vi "WriteToGlobalsFromNT.vi"() -> ()   [LabVIEW 2019]
uses:
  <vilib>/Rock Robotics/Network Tables/NT Read String Array.vi
  CalibrationsGlobalVariables.vi
panel:
  in  "ControlPanelArray":string[](array[string])=["Spinwheel_Throttle", "time_to_run"]
  in  "MagazineArray":string[](array[string])=["Top_IR_Threshold", "Top_Middle_IR_Threshold", "Bottom_Middle_IR_Threshold", "Bottom_IR_Threshold", "Loading_Speed", "Firing_Speed", "Unjam_Speed", "Max_Magazine_Speed"]
  in  "IntakeArray":string[](array[string])=["retract_delay(ms)", "extend_delay(ms)", "Intake Input", "Hopper Input", "Intake_Speed"]
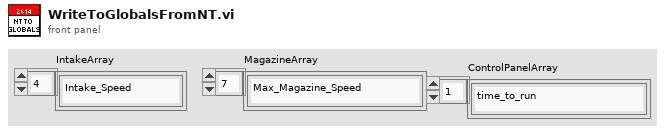
[diagram p1: front panel]
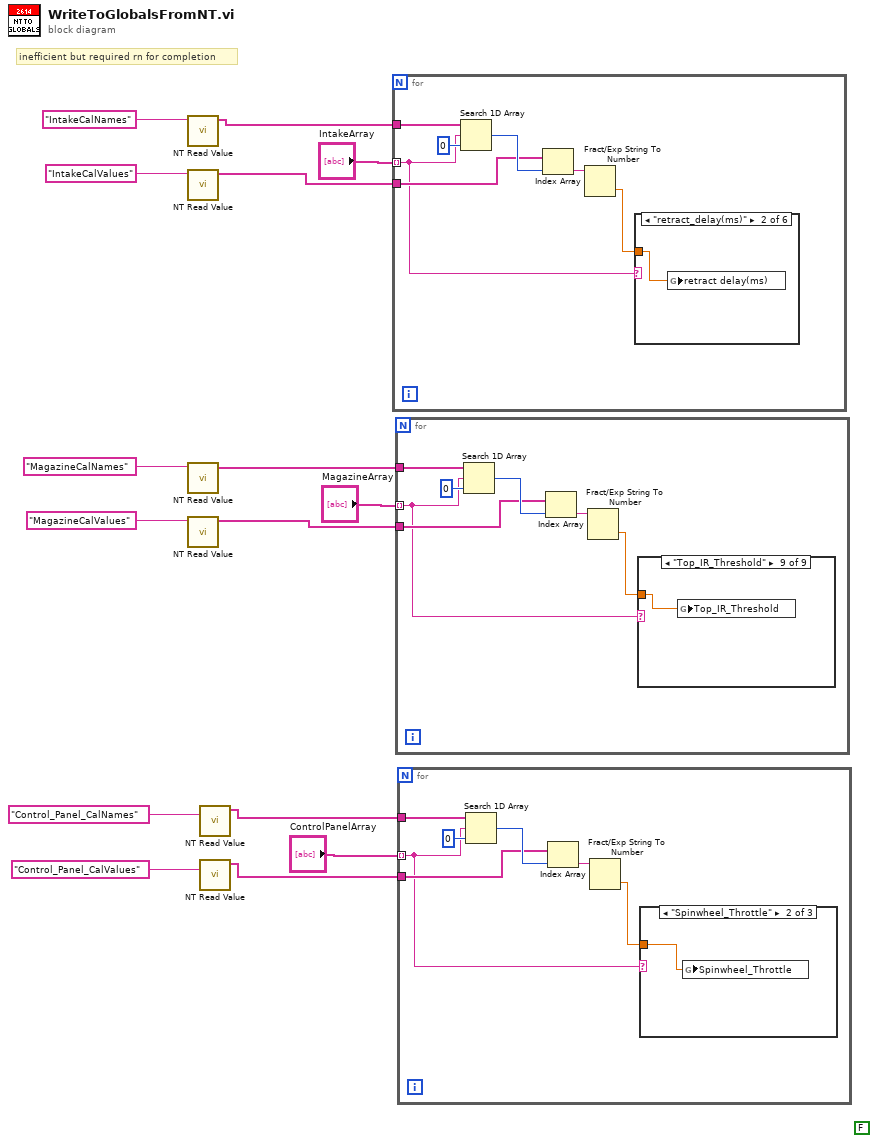
[diagram p0: block diagram]
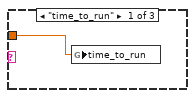
[diagram p2: hidden frame]
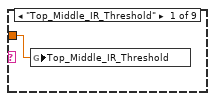
[diagram p4: hidden frame]
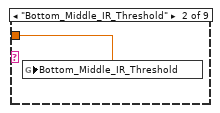
[diagram p5: hidden frame]
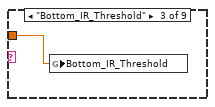
[diagram p6: hidden frame]
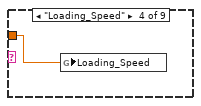
[diagram p7: hidden frame]
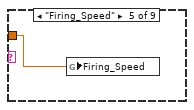
[diagram p8: hidden frame]
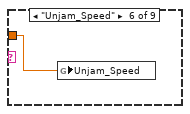
[diagram p9: hidden frame]
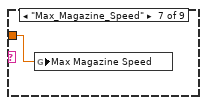
[diagram p10: hidden frame]
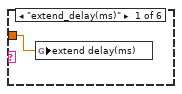
[diagram p12: hidden frame]
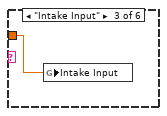
[diagram p13: hidden frame]
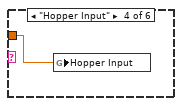
[diagram p14: hidden frame]
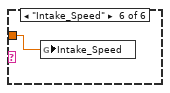
[diagram p16: hidden frame]
diagram:
  (unwired) FALSE
  # "inefficient but required rn for completion"
  n1 = call-poly <vilib>:"NT Read Value.vi"("Name"="IntakeCalNames") -> ("String Array"=w8:string[])  [unwired: 9 in, 1 out]
  n2 = call-poly <vilib>:"NT Read Value.vi"("Name"="IntakeCalValues") -> ("String Array"=w9:string[])  [unwired: 9 in, 1 out]
  n3 = call-poly <vilib>:"NT Read Value.vi"("Name"="MagazineCalNames") -> ("String Array"=w5:string[])  [unwired: 9 in, 1 out]
  n4 = call-poly <vilib>:"NT Read Value.vi"("Name"="MagazineCalValues") -> ("String Array"=w4:string[])  [unwired: 9 in, 1 out]
  n5 = call-poly <vilib>:"NT Read Value.vi"("Name"="Control_Panel_CalNames") -> ("String Array"=w3:string[])  [unwired: 9 in, 1 out]
  n6 = call-poly <vilib>:"NT Read Value.vi"("Name"="Control_Panel_CalValues") -> ("String Array"=w2:string[])  [unwired: 9 in, 1 out]
  n7 = for {
    tunnel: w9 -> [w19]
    tunnel: w8 -> [w18]
    tunnel: "IntakeArray" -> [w17] mode=indexing
    n8 = Search 1D Array(1D array=w18, element=w17, start index (0)=0) -> (index of element=w21:i32)
    n9 = Index Array(array=w19, index=w21) -> (element=w20:string)
    n10 = Fract/Exp String To Number(string=w20) -> (number=w16:dbl)  [unwired: 3 in, 1 out]
    n11 = case shown="\"retract_delay(ms)\"" w17 {
      tunnel: w16 -> [w23 w24 w25 w26 _ w27]
      frame "extend_delay(ms)" {
        n12 = global write "CalibrationsGlobalVariables.vi" "extend delay(ms)"(w23) -> ()
      }
      frame "retract_delay(ms)" {
        n13 = global write "CalibrationsGlobalVariables.vi" "retract delay(ms)"(w24) -> ()
      }
      frame "Intake Input" {
        n14 = global write "CalibrationsGlobalVariables.vi" "Intake Input"(w25) -> ()
      }
      frame "Hopper Input" {
        n15 = global write "CalibrationsGlobalVariables.vi" "Hopper Input"(w26) -> ()
      }
      frame "", Default {
      }
      frame "Intake_Speed" {
        n16 = global write "CalibrationsGlobalVariables.vi" "Intake_Speed"(w27) -> ()
      }
    }
  }
  n17 = for {
    tunnel: w4 -> [w31]
    tunnel: w5 -> [w30]
    tunnel: "MagazineArray" -> [w29] mode=indexing
    n18 = Search 1D Array(1D array=w30, element=w29, start index (0)=0) -> (index of element=w33:i32)
    n19 = Index Array(array=w31, index=w33) -> (element=w32:string)
    n20 = Fract/Exp String To Number(string=w32) -> (number=w28:dbl)  [unwired: 3 in, 1 out]
    n21 = case shown="\"Top_IR_Threshold\"" w29 {
      tunnel: w28 -> [w35 w36 w37 w38 w39 w40 w41 _ w42]
      frame "Top_Middle_IR_Threshold" {
        n22 = global write "CalibrationsGlobalVariables.vi" "Top_Middle_IR_Threshold"(w35) -> ()
      }
      frame "Bottom_Middle_IR_Threshold" {
        n23 = global write "CalibrationsGlobalVariables.vi" "Bottom_Middle_IR_Threshold"(w36) -> ()
      }
      frame "Bottom_IR_Threshold" {
        n24 = global write "CalibrationsGlobalVariables.vi" "Bottom_IR_Threshold"(w37) -> ()
      }
      frame "Loading_Speed" {
        n25 = global write "CalibrationsGlobalVariables.vi" "Loading_Speed"(w38) -> ()
      }
      frame "Firing_Speed" {
        n26 = global write "CalibrationsGlobalVariables.vi" "Firing_Speed"(w39) -> ()
      }
      frame "Unjam_Speed" {
        n27 = global write "CalibrationsGlobalVariables.vi" "Unjam_Speed"(w40) -> ()
      }
      frame "Max_Magazine_Speed" {
        n28 = global write "CalibrationsGlobalVariables.vi" "Max Magazine Speed"(w41) -> ()
      }
      frame "", Default {
      }
      frame "Top_IR_Threshold" {
        n29 = global write "CalibrationsGlobalVariables.vi" "Top_IR_Threshold"(w42) -> ()
      }
    }
  }
  n30 = for {
    tunnel: w2 -> [w46]
    tunnel: w3 -> [w45]
    tunnel: "ControlPanelArray" -> [w44] mode=indexing
    n31 = Search 1D Array(1D array=w45, element=w44, start index (0)=0) -> (index of element=w48:i32)
    n32 = Index Array(array=w46, index=w48) -> (element=w47:string)
    n33 = Fract/Exp String To Number(string=w47) -> (number=w43:dbl)  [unwired: 3 in, 1 out]
    n34 = case shown="\"Spinwheel_Throttle\"" w44 {
      tunnel: w43 -> [w50 w51 _]
      frame "time_to_run" {
        n35 = global write "CalibrationsGlobalVariables.vi" "time_to_run"(w50) -> ()
      }
      frame "Spinwheel_Throttle" {
        n36 = global write "CalibrationsGlobalVariables.vi" "Spinwheel_Throttle"(w51) -> ()
      }
      frame "", Default {
      }
    }
  }
